vi "nanocal -- nuclear schottky fit V3.vi"() -> ()   [LabVIEW 2020] (continued)
\"mm1\"-> 0.000103608352  , \"mm2\"-> 0.017542867394  , \"mm3\"-> 0.085978401835  , \"T\"->  0.300000000000  , \"B\"-> 12.000000000000  , \"θ\"-> 90.000000000000  |>   , \r76 ->   <| \"ζ\"->  0.044154556051  , \"τ1\"-> 0.038823125235  , \"τS\"-> 0.027069314930  , \"τN\"-> 0.013601990730  , \"τC\"-> 0.002287979276  , \"κ0\"-> 0.000000002359  , \"mm1\"-> 0.000089763345  , \"mm2\"-> 0.018083678254  , \"mm3\"-> 0.065404792018  , \"T\"->  0.360000000000  , \"B\"-> 12.000000000000  , \"θ\"-> 90.000000000000  |>   , \r77 ->   <| \"ζ\"->  0.032748569996  , \"τ1\"-> 0.031072007290  , \"τS\"-> 0.024343937548  , \"τN\"-> 0.006961654481  , \"τC\"-> 0.002967111565  , \"κ0\"-> 0.000000002964  , \"mm1\"-> 0.000084402249  , \"mm2\"-> 0.018055855929  , \"mm3\"-> 0.048229666078  , \"T\"->  0.430000000000  , \"B\"-> 12.000000000000  , \"θ\"-> 90.000000000000  |>   , \r78 ->   <| \"ζ\"->  0.027599263457  , \"τ1\"-> 0.026239105728  , \"τS\"-> 0.022370859308  , \"τN\"-> 0.003857632966  , \"τC\"-> 0.003499360499  , \"κ0\"-> 0.000000003681  , \"mm1\"-> 0.000081816106  , \"mm2\"-> 0.017901054668  , \"mm3\"-> 0.038707974796  , \"T\"->  0.512000000000  , \"B\"-> 12.000000000000  , \"θ\"-> 90.000000000000  |>   , \r79 ->   <| \"ζ\"->  0.020568815513  , \"τ1\"-> 0.023045965648  , \"τS\"-> 0.020791387386  , \"τN\"-> 0.002229171297  , \"τC\"-> 0.004427475438  , \"κ0\"-> 0.000000004398  , \"mm1\"-> 0.000074037290  , \"mm2\"-> 0.017820522459  , \"mm3\"-> 0.033072945644  , \"T\"->  0.610000000000  , \"B\"-> 12.000000000000  , \"θ\"-> 90.000000000000  |>   , \r80 ->   <| \"ζ\"->  0.016159836955  , \"τ1\"-> 0.019958638777  , \"τS\"-> 0.018730096307  , \"τN\"-> 0.000899236968  , \"τC\"-> 0.005152267403  , \"κ0\"-> 0.000000006087  , \"mm1\"-> 0.000064651231  , \"mm2\"-> 0.017530317649  , \"mm3\"-> 0.027462477400  , \"T\"->  0.810000000000  , \"B\"-> 12.000000000000  , \"θ\"-> 90.000000000000  |>   , \r81 ->   <| \"ζ\"->  0.014495870556  , \"τ1\"-> 0.019990087457  , \"τS\"-> 0.016832201384  , \"τN\"-> 0.000455517238  , \"τC\"-> 0.005555782498  , \"κ0\"-> 0.000000008420  , \"mm1\"-> 0.000060055560  , \"mm2\"-> 0.018114231010  , \"mm3\"-> 0.024909902538  , \"T\"->  1.100000000000  , \"B\"-> 12.000000000000  , \"θ\"-> 90.000000000000  |>   , \r82 ->   <| \"ζ\"->  0.014043763709  , \"τ1\"-> 0.018292068543  , \"τS\"-> 0.011311396743  , \"τN\"-> 0.000128802259  , \"τC\"-> 0.008087849636  , \"κ0\"-> 0.000000014258  , \"mm1\"-> 0.000065912054  , \"mm2\"-> 0.017276417784  , \"mm3\"-> 0.020638450794  , \"T\"->  1.800000000000  , \"B\"-> 12.000000000000  , \"θ\"-> 90.000000000000  |>   , \r83 ->   <| \"ζ\"->  0.016187684631  , \"τ1\"-> 0.018325345271  , \"τS\"-> 0.007510087776  , \"τN\"-> 0.000028419157  , \"τC\"-> 0.008115463080  , \"κ0\"-> 0.000000024747  , \"mm1\"-> 0.000062903858  , \"mm2\"-> 0.015524812312  , \"mm3\"-> 0.018513630087  , \"T\"->  3.000000000000  , \"B\"-> 12.000000000000  , \"θ\"-> 90.000000000000  |>   , \r84 ->   <| \"ζ\"->  0.027897403691  , \"τ1\"-> 0.014639690770  , \"τS\"-> 0.004105291179  , \"τN\"-> 0.000006999171  , \"τC\"-> 0.007414449545  , \"κ0\"-> 0.000000059701  , \"mm1\"-> 0.000073450671  , \"mm2\"-> 0.011534391407  , \"mm3\"-> 0.014673310811  , \"T\"->  5.700000000000  , \"B\"-> 12.000000000000  , \"θ\"-> 90.000000000000  |>   , \r"
  out "filenames":map{i32, string}(c390)={4026="CeCoIn5_3rd_4026_ref_12T_0.127K_60deg_changeT_fsweep_labview_.dat", 4027="CeCoIn5_3rd_4027_ref_12T_0.15K_60deg_changeT_fsweep_labview_.dat", 4028="CeCoIn5_3rd_4028_ref_12T_0.179K_60deg_changeT_fsweep_labview_.dat", 4029="CeCoIn5_3rd_4029_ref_12T_0.20K_60deg_changeT_fsweep_labview_.dat", 4030="CeCoIn5_3rd_4030_ref_12T_0.24K_60deg_changeT_fsweep_labview_.dat", 4031="CeCoIn5_3rd_4031_ref_12T_0.287K_60deg_changeT_fsweep_labview_.dat", 4032="CeCoIn5_3rd_4032_ref_12T_0.33K_60deg_changeT_fsweep_labview_.dat", 4033="CeCoIn5_3rd_4033_ref_12T_0.43K_60deg_changeT_fsweep_labview_.dat", 4034="CeCoIn5_3rd_4034_ref_12T_0.51K_60deg_changeT_fsweep_labview_.dat", 4035="CeCoIn5_3rd_4035_ref_12T_0.62K_60deg_changeT_fsweep_labview_.dat", 4036="CeCoIn5_3rd_4036_ref_12T_0.83K_60deg_changeT_fsweep_labview_.dat", 4037="CeCoIn5_3rd_4037_ref_12T_1.13K_60deg_changeT_fsweep_labview_.dat", 4038="CeCoIn5_3rd_4038_ref_12T_1.90K_60deg_changeT_fsweep_labview_.dat", 4039="CeCoIn5_3rd_4039_ref_12T_3.15K_60deg_changeT_fsweep_labview_.dat", 4040="CeCoIn5_3rd_4040_ref_12T_5.70K_60deg_changeT_fsweep_labview_.dat", 4041="CeCoIn5_3rd_4041_ref_12T_7.87K_60deg_changeT_fsweep_labview_.dat", 4042="CeCoIn5_3rd_4042_ref_12T_9.80K_60deg_changeT_fsweep_labview_.dat", 4043="CeCoIn5_3rd_4043_ref_12T_12.36K_60deg_changeT_fsweep_labview_.dat", 4044="CeCoIn5_3rd_4044_ref_12T_14.80K_60deg_changeT_fsweep_labview_.dat", 4045="CeCoIn5_3rd_4045_ref_12T_16.42K_60deg_changeT_fsweep_labview_.dat", 4046="CeCoIn5_3rd_4046_ref_12T_18.04K_60deg_changeT_fsweep_labview_.dat", 4047="CeCoIn5_2nd_4047_12T_ref_0.14K_0deg_changeT_fsweep_labview_.dat", 4048="CeCoIn5_2nd_4048_12T_ref_0.17K_0deg_changeT_fsweep_labview_.dat", 4049="CeCoIn5_2nd_4049_12T_ref_0.20K_0deg_changeT_fsweep_labview_.dat", 4050="CeCoIn5_2nd_4050_12T_ref_0.22K_0deg_changeT_fsweep_labview_.dat", 4051="CeCoIn5_2nd_4051_12T_ref_0.28K_0deg_changeT_fsweep_labview_.dat", 4052="CeCoIn5_2nd_4052_12T_ref_0.33K_0deg_changeT_fsweep_labview_.dat", 4053="CeCoIn5_2nd_4053_12T_ref_0.40K_0deg_changeT_fsweep_labview_.dat", 4054="CeCoIn5_2nd_4054_12T_ref_0.48K_0deg_changeT_fsweep_labview_.dat", 4055="CeCoIn5_2nd_4055_12T_ref_0.58K_0deg_changeT_fsweep_labview_.dat", 4056="CeCoIn5_2nd_4056_12T_ref_0.68K_0deg_changeT_fsweep_labview_.dat", 4057="CeCoIn5_2nd_4057_12T_ref_0.91K_0deg_changeT_fsweep_labview_.dat", 4058="CeCoIn5_2nd_4058_12T_ref_1.23K_0deg_changeT_fsweep_labview_.dat", 4059="CeCoIn5_2nd_4059_12T_ref_1.97K_0deg_changeT_fsweep_labview_.dat", 4060="CeCoIn5_2nd_4060_12T_ref_3.19K_0deg_changeT_fsweep_labview_.dat", 4061="CeCoIn5_2nd_4061_12T_ref_5.82K_0deg_changeT_fsweep_labview_.dat", 4070="CeCoIn5_2nd_4070_12T_ref_0.20K_90deg_changeT_fsweep_labview_.dat", 4071="CeCoIn5_2nd_4071_12T_ref_0.14K_90deg_changeT_fsweep_labview_.dat", 4072="CeCoIn5_2nd_4072_12T_ref_0.18K_90deg_changeT_fsweep_labview_.dat", 4073="CeCoIn5_2nd_4073_12T_ref_0.22K_90deg_changeT_fsweep_labview_.dat", 4074="CeCoIn5_2nd_4074_12T_ref_0.27K_90deg_changeT_fsweep_labview_.dat", 4075="CeCoIn5_2nd_4075_12T_ref_0.33K_90deg_changeT_fsweep_labview_.dat", 4076="CeCoIn5_2nd_4076_12T_ref_0.39K_90deg_changeT_fsweep_labview_.dat", 4077="CeCoIn5_2nd_4077_12T_ref_0.48K_90deg_changeT_fsweep_labview_.dat", 4078="CeCoIn5_2nd_4078_12T_ref_0.58K_90deg_changeT_fsweep_labview_.dat", 4079="CeCoIn5_2nd_4079_12T_ref_0.68K_90deg_changeT_fsweep_labview_.dat", 4080="CeCoIn5_2nd_4080_12T_ref_0.91K_90deg_changeT_fsweep_labview_.dat", 4081="CeCoIn5_2nd_4081_12T_ref_1.23K_90deg_changeT_fsweep_labview_.dat", 4082="CeCoIn5_2nd_4082_12T_ref_2.05K_90deg_changeT_fsweep_labview_.dat", 4083="CeCoIn5_2nd_4083_12T_ref_3.31K_90deg_changeT_fsweep_labview_.dat", 4084="CeCoIn5_2nd_4084_12T_ref_6.0K_90deg_changeT_fsweep_labview_.dat", 4094="CeCoIn5_2nd_4094_6T_0.30K_90deg_ref_changeB_fsweep_labview_.dat", 4095="CeCoIn5_2nd_4095_6T_0.197K_90deg_ref_changeB_fsweep_labview_.dat", 4098="CeCoIn5_2nd_4098_6T_0.148K_90deg_ref_changeB_fsweep_labview_.dat", 4099="CeCoIn5_2nd_4099_9T_0.197K_90deg_ref_changeB_fsweep_labview_.dat", 4100="CeCoIn5_2nd_4100_11T_0.197K_90deg_ref_changeB_fsweep_labview_.dat", 4101="CeCoIn5_2nd_4101_10T_0.197K_90deg_ref_changeB_fsweep_labview_.dat", 4102="CeCoIn5_2nd_4102_8T_0.197K_90deg_ref_changeB_fsweep_labview_.dat", 4103="CeCoIn5_2nd_4103_7T_0.197K_90deg_ref_changeB_fsweep_labview_.dat", 4104="CeCoIn5_2nd_4104_5T_0.197K_90deg_ref_changeB_fsweep_labview_.dat", 4105="CeCoIn5_2nd_4105_0T_0.197K_90deg_ref_changeB_fsweep_labview_.dat", 4106="CeCoIn5_2nd_4106_0T_1.55K_90deg_ref_changeB_fsweep_labview_.dat", 4107="CeCoIn5_2nd_4107_0T_1.00K_90deg_ref_changeB_fsweep_labview_.dat", 4108="CeCoIn5_2nd_4108_0T_0.67K_90deg_ref_changeB_fsweep_labview_.dat", 4110="CeCoIn5_4th_4110_ref_12T_0.16K_30deg_changeT_fsweep_labview_.dat", 4112="CeCoIn5_4th_4112_ref_12T_0.17K_30deg_changeT_fsweep_labview_.dat", 4113="CeCoIn5_4th_4113_ref_12T_0.14K_30deg_changeT_fsweep_labview_.dat", 4114="CeCoIn5_4th_4114_ref_12T_0.20K_30deg_changeT_fsweep_labview_.dat", 4115="CeCoIn5_4th_4115_ref_12T_0.25K_30deg_changeT_fsweep_labview_.dat", 4116="CeCoIn5_4th_4116_ref_12T_0.30K_30deg_changeT_fsweep_labview_.dat", 4117="CeCoIn5_4th_4117_ref_12T_0.36K_30deg_changeT_fsweep_labview_.dat", 4118="CeCoIn5_4th_4118_ref_12T_0.43K_30deg_changeT_fsweep_labview_.dat", 4119="CeCoIn5_4th_4119_ref_12T_0.53K_30deg_changeT_fsweep_labview_.dat", 4120="CeCoIn5_4th_4120_ref_12T_0.62K_30deg_changeT_fsweep_labview_.dat", 4121="CeCoIn5_4th_4121_ref_12T_0.83K_30deg_changeT_fsweep_labview_.dat", 4122="CeCoIn5_4th_4122_ref_12T_1.13K_30deg_changeT_fsweep_labview_.dat", 4123="CeCoIn5_4th_4123_ref_12T_1.90K_30deg_changeT_fsweep_labview_.dat", 4124="CeCoIn5_4th_4124_ref_12T_3.10K_30deg_changeT_fsweep_labview_.dat", 8026="CeCoIn5_3rd_8026_sam_12T_0.127K_60deg_changeT_fsweep_labview_.dat", 8027="CeCoIn5_3rd_8027_sam_12T_0.15K_60deg_changeT_fsweep_labview_.dat", 8028="CeCoIn5_3rd_8028_sam_12T_0.179K_60deg_changeT_fsweep_labview_.dat", 8029="CeCoIn5_3rd_8029_sam_12T_0.20K_60deg_changeT_fsweep_labview_.dat", 8030="CeCoIn5_3rd_8030_sam_12T_0.24K_60deg_changeT_fsweep_labview_.dat", 8031="CeCoIn5_3rd_8031_sam_12T_0.287K_60deg_changeT_fsweep_labview_.dat", 8032="CeCoIn5_3rd_8032_sam_12T_0.33K_60deg_changeT_fsweep_labview_.dat", 8033="CeCoIn5_3rd_8033_sam_12T_0.43K_60deg_changeT_fsweep_labview_.dat", 8034="CeCoIn5_3rd_8034_sam_12T_0.51K_60deg_changeT_fsweep_labview_.dat", 8035="CeCoIn5_3rd_8035_sam_12T_0.62K_60deg_changeT_fsweep_labview_.dat", 8036="CeCoIn5_3rd_8036_sam_12T_0.83K_60deg_changeT_fsweep_labview_.dat", 8037="CeCoIn5_3rd_8037_sam_12T_1.13K_60deg_changeT_fsweep_labview_.dat", 8038="CeCoIn5_3rd_8038_sam_12T_1.90K_60deg_changeT_fsweep_labview_.dat", 8039="CeCoIn5_3rd_8039_sam_12T_3.15K_60deg_changeT_fsweep_labview_.dat", 8040="CeCoIn5_3rd_8040_sam_12T_5.70K_60deg_changeT_fsweep_labview_.dat", 8041="CeCoIn5_3rd_8041_sam_12T_7.87K_60deg_changeT_fsweep_labview_.dat", 8042="CeCoIn5_3rd_8042_sam_12T_9.80K_60deg_changeT_fsweep_labview_.dat", 8043="CeCoIn5_3rd_8043_sam_12T_12.36K_60deg_changeT_fsweep_labview_.dat", 8044="CeCoIn5_3rd_8044_sam_12T_14.80K_60deg_changeT_fsweep_labview_.dat", 8045="CeCoIn5_3rd_8045_sam_12T_16.42K_60deg_changeT_fsweep_labview_.dat", 8046="CeCoIn5_3rd_8046_sam_12T_18.04K_60deg_changeT_fsweep_labview_.dat", 8047="CeCoIn5_2nd_8047_12T_sam_0.12K_0deg_changeT_fsweep_labview_.dat", 8048="CeCoIn5_2nd_8048_12T_sam_0.148K_0deg_changeT_fsweep_labview_.dat", 8049="CeCoIn5_2nd_8049_12T_sam_0.179K_0deg_changeT_fsweep_labview_.dat", 8050="CeCoIn5_2nd_8050_12T_sam_0.197K_0deg_changeT_fsweep_labview_.dat", 8051="CeCoIn5_2nd_8051_12T_sam_0.25K_0deg_changeT_fsweep_labview_.dat", 8052="CeCoIn5_2nd_8052_12T_sam_0.3K_0deg_changeT_fsweep_labview_.dat", 8053="CeCoIn5_2nd_8053_12T_sam_0.360K_0deg_changeT_fsweep_labview_.dat", 8054="CeCoIn5_2nd_8054_12T_sam_0.430K_0deg_changeT_fsweep_labview_.dat", 8055="CeCoIn5_2nd_8055_12T_sam_0.512K_0deg_changeT_fsweep_labview_.dat", 8056="CeCoIn5_2nd_8056_12T_sam_0.61K_0deg_changeT_fsweep_labview_.dat", 8057="CeCoIn5_2nd_8057_12T_sam_0.81K_0deg_changeT_fsweep_labview_.dat", 8058="CeCoIn5_2nd_8058_12T_sam_1.12K_0deg_changeT_fsweep_labview_.dat", 8059="CeCoIn5_2nd_8059_12T_sam_1.8K_0deg_changeT_fsweep_labview_.dat", 8060="CeCoIn5_2nd_8060_12T_sam_3.0K_0deg_changeT_fsweep_labview_.dat", 8061="CeCoIn5_2nd_8061_12T_sam_5.5K_0deg_changeT_fsweep_labview_.dat", 8070="CeCoIn5_2nd_8070_12T_sam_0.179K_90deg_changeT_fsweep_labview_.dat", 8071="CeCoIn5_2nd_8071_12T_sam_0.120K_90deg_changeT_fsweep_labview_.dat", 8072="CeCoIn5_2nd_8072_12T_sam_0.148K_90deg_changeT_fsweep_labview_.dat", 8073="CeCoIn5_2nd_8073_12T_sam_0.197K_90deg_changeT_fsweep_labview_.dat", 8074="CeCoIn5_2nd_8074_12T_sam_0.249K_90deg_changeT_fsweep_labview_.dat", 8075="CeCoIn5_2nd_8075_12T_sam_0.300K_90deg_changeT_fsweep_labview_.dat", 8076="CeCoIn5_2nd_8076_12T_sam_0.360K_90deg_changeT_fsweep_labview_.dat", 8077="CeCoIn5_2nd_8077_12T_sam_0.430K_90deg_changeT_fsweep_labview_.dat", 8078="CeCoIn5_2nd_8078_12T_sam_0.512K_90deg_changeT_fsweep_labview_.dat", 8079="CeCoIn5_2nd_8079_12T_sam_0.610K_90deg_changeT_fsweep_labview_.dat", 8080="CeCoIn5_2nd_8080_12T_sam_0.810K_90deg_changeT_fsweep_labview_.dat", 8081="CeCoIn5_2nd_8081_12T_sam_1.1K_90deg_changeT_fsweep_labview_.dat", 8082="CeCoIn5_2nd_8082_12T_sam_1.8K_90deg_changeT_fsweep_labview_.dat", 8083="CeCoIn5_2nd_8083_12T_sam_3.0K_90deg_changeT_fsweep_labview_.dat", 8084="CeCoIn5_2nd_8084_12T_sam_5.7K_90deg_changeT_fsweep_labview_.dat", 8094="CeCoIn5_2nd_8094_6T_0.30K_90deg_sam_changeB_fsweep_labview_.dat", 8095="CeCoIn5_2nd_8095_6T_0.197K_90deg_sam_changeB_fsweep_labview_.dat", 8098="CeCoIn5_2nd_8098_6T_0.148K_90deg_sam_changeB_fsweep_labview_.dat", 8099="CeCoIn5_2nd_8099_9T_0.197K_90deg_sam_changeB_fsweep_labview_.dat", 8100="CeCoIn5_2nd_8100_11T_0.197K_90deg_sam_changeB_fsweep_labview_.dat", 8101="CeCoIn5_2nd_8101_10T_0.197K_90deg_sam_changeB_fsweep_labview_.dat", 8102="CeCoIn5_2nd_8102_8T_0.197K_90deg_sam_changeB_fsweep_labview_.dat", 8103="CeCoIn5_2nd_8103_7T_0.197K_90deg_sam_changeB_fsweep_labview_.dat", 8104="CeCoIn5_2nd_8104_5T_0.197K_90deg_sam_changeB_fsweep_labview_.dat", 8105="CeCoIn5_2nd_8105_0T_0.197K_90deg_sam_changeB_fsweep_labview_.dat", 8106="CeCoIn5_2nd_8106_0T_1.55K_90deg_sam_changeB_fsweep_labview_.dat", 8107="CeCoIn5_2nd_8107_0T_1.00K_90deg_sam_changeB_fsweep_labview_.dat", 8108="CeCoIn5_2nd_8108_0T_0.67K_90deg_sam_changeB_fsweep_labview_.dat", 8110="CeCoIn5_4th_8110_sam_12T_0.16K_30deg_changeT_fsweep_labview_.dat", 8112="CeCoIn5_4th_8112_sam_12T_0.17K_30deg_changeT_fsweep_labview_.dat", 8113="CeCoIn5_4th_8113_sam_12T_0.14K_30deg_changeT_fsweep_labview_.dat", 8114="CeCoIn5_4th_8114_sam_12T_0.20K_30deg_changeT_fsweep_labview_.dat", 8115="CeCoIn5_4th_8115_sam_12T_0.25K_30deg_changeT_fsweep_labview_.dat", 8116="CeCoIn5_4th_8116_sam_12T_0.30K_30deg_changeT_fsweep_labview_.dat", 8117="CeCoIn5_4th_8117_sam_12T_0.36K_30deg_changeT_fsweep_labview_.dat", 8118="CeCoIn5_4th_8118_sam_12T_0.43K_30deg_changeT_fsweep_labview_.dat", 8119="CeCoIn5_4th_8119_sam_12T_0.53K_30deg_changeT_fsweep_labview_.dat", 8120="CeCoIn5_4th_8120_sam_12T_0.62K_30deg_changeT_fsweep_labview_.dat", 8121="CeCoIn5_4th_8121_sam_12T_0.83K_30deg_changeT_fsweep_labview_.dat", 8122="CeCoIn5_4th_8122_sam_12T_1.13K_30deg_changeT_fsweep_labview_.dat", 8123="CeCoIn5_4th_8123_sam_12T_1.90K_30deg_changeT_fsweep_labview_.dat", 8124="CeCoIn5_4th_8124_sam_12T_3.10K_30deg_changeT_fsweep_labview_.dat", 40047="CeCoIn5_3rd_40047_ref_12T_19.60K_60deg_changeT_fsweep_labview_.dat", 40049="CeCoIn5_3rd_40049_ref_12T_0.129K_60deg_changeT_fsweep_labview_.dat", 40125="CeCoIn5_4th___40125__(039)__C(f)_12T_0.157K_45deg _changeT_ref_fromraw__labview_.dat", 40126="CeCoIn5_4th___40126__(040)__C(f)_12T_0.120K_45deg_changeT_ref_fromraw__labview_.dat", 40127="CeCoIn5_4th___40127__(041)__C(f)_12T_0.170K_45deg_changeT_ref_fromraw__labview_.dat", 40128="CeCoIn5_4th___40128__(042)__C(f)_12T_0.200K_45deg_changeT_ref_fromraw__labview_.dat", 40129="CeCoIn5_4th___40129__(043)__C(f)_12T_0.255K_45deg_changeT_ref_fromraw__labview_.dat", 40130="CeCoIn5_4th___40130__(044)__C(f)_12T_0.300K_45deg_changeT_ref_fromraw__labview_.dat", 40131="CeCoIn5_4th___40131__(045)__C(f)_12T_0.360K_45deg_changeT_ref_fromraw__labview_.dat", 40132="CeCoIn5_4th___40132__(046)__C(f)_12T_0.43K_45deg_changeT_ref_fromraw__labview_.dat", 40133="CeCoIn5_4th___40133__(047)__C(f)_12T_0.53K_45deg_changeT_ref_fromraw__labview_.dat", 40134="CeCoIn5_4th___40134__(048)__C(f)_12T_0.62K_45deg_changeT_ref_fromraw__labview_.dat", 40135="CeCoIn5_4th___40135__(049)__C(f)_12T_0.83K_45deg_changeT_ref_fromraw__labview_.dat", 40136="CeCoIn5_4th___40136__(050)__C(f)_12T_1.13K_45deg_changeT_ref_fromraw__labview_.dat", 40137="CeCoIn5_4th___40137__(051)__C(f)_12T_1.90K_45deg_changeT_ref_fromraw__labview_.dat", 40138="CeCoIn5_4th___40138__(052)__C(f)_12T_3.10K_45deg_changeT_ref_fromraw__labview_.dat", 40139="CeCoIn5_4th___40139__(053)__C(f)_12T_5.70K_45deg_changeT_ref_fromraw__labview_.dat", 80047="CeCoIn5_3rd_80047_sam_12T_19.60K_60deg_changeT_fsweep_labview_.dat", 80049="CeCoIn5_3rd_80049_sam_12T_0.129K_60deg_changeT_fsweep_labview_.dat", 80125="CeCoIn5_4th___80125__(039)__C(f)_12T_0.157K_45deg _changeT_sam_fromraw__labview_.dat", 80126="CeCoIn5_4th___80126__(040)__C(f)_12T_0.120K_45deg_changeT_sam_fromraw__labview_.dat", 80127="CeCoIn5_4th___80127__(041)__C(f)_12T_0.170K_45deg_changeT_sam_fromraw__labview_.dat", 80128="CeCoIn5_4th___80128__(042)__C(f)_12T_0.200K_45deg_changeT_sam_fromraw__labview_.dat", 80129="CeCoIn5_4th___80129__(043)__C(f)_12T_0.255K_45deg_changeT_sam_fromraw__labview_.dat", 80130="CeCoIn5_4th___80130__(044)__C(f)_12T_0.300K_45deg_changeT_sam_fromraw__labview_.dat", 80131="CeCoIn5_4th___80131__(045)__C(f)_12T_0.360K_45deg_changeT_sam_fromraw__labview_.dat", 80132="CeCoIn5_4th___80132__(046)__C(f)_12T_0.43K_45deg_changeT_sam_fromraw__labview_.dat", 80133="CeCoIn5_4th___80133__(047)__C(f)_12T_0.53K_45deg_changeT_sam_fromraw__labview_.dat", 80134="CeCoIn5_4th___80134__(048)__C(f)_12T_0.62K_45deg_changeT_sam_fromraw__labview_.dat", 80135="CeCoIn5_4th___80135__(049)__C(f)_12T_0.83K_45deg_changeT_sam_fromraw__labview_.dat", 80136="CeCoIn5_4th___80136__(050)__C(f)_12T_1.13K_45deg_changeT_sam_fromraw__labview_.dat", 80137="CeCoIn5_4th___80137__(051)__C(f)_12T_1.90K_45deg_changeT_sam_fromraw__labview_.dat", 80138="CeCoIn5_4th___80138__(052)__C(f)_12T_3.10K_45deg_changeT_sam_fromraw__labview_.dat", 80139="CeCoIn5_4th___80139__(053)__C(f)_12T_5.70K_45deg_changeT_sam_fromraw__labview_.dat"}
  out "constrained filename lookup":map{i32, i32}(c390)={0=40126, 1=40125, 2=40127, 3=40128, 4=40129, 5=40130, 6=40131, 7=40132, 8=40133, 9=40134, 10=40135, 11=40136, 12=40137, 13=40138, 14=40139}
  out "Set of B's":set{dbl}(c389)={0.0, 5.0, 6.0, 7.0, 8.0, 9.0, 10.0, 11.0, 12.0}
  out "Set of θ's":set{dbl}(c389)={0.0, 30.0, 45.0, 60.0, 90.0}
  out "Set of T's":set{dbl}(c389)={0.12, 0.127, 0.129, 0.14, 0.148, 0.15, 0.157, 0.16, 0.17, 0.179, 0.18, 0.197, 0.2, 0.22, 0.24, 0.249, 0.25, 0.255, 0.27, 0.28, 0.287, 0.3, 0.33, 0.36, 0.39, 0.4, 0.43, 0.48, 0.51, 0.512, 0.53, 0.58, 0.61, 0.62, 0.67, 0.68, 0.81, 0.83, 0.91, 1.0, 1.1, 1.12, 1.13, 1.23, 1.55, 1.8, 1.9, 1.97, 2.05, 3.0, 3.1, 3.15, 3.19, 3.31, 5.5, 5.7, 5.82, 6.0, 7.87, 9.8, 12.36, 14.8, 16.42, 18.04, 19.6}
  out "B lookup":map{i32, dbl}(c390)={0=0.0, 1=5.0, 2=6.0, 3=7.0, 4=8.0, 5=9.0, 6=10.0, 7=11.0, 8=12.0}
  out "filesnames lookup":map{i32, i32}(c390)={0=8047, 1=8071, 2=40126, 3=80126, 4=4026, 5=8026, 6=40049, 7=80049, 8=4047, 9=4071, 10=4113, 11=8113, 12=4098, 13=8048, 14=8072, 15=8098, 16=4027, 17=8027, 18=40125, 19=80125, 20=4110, 21=8110, 22=4048, 23=4112, 24=8112, 25=40127, 26=80127, 27=4028, 28=8028, 29=8049, 30=8070, 31=4072, 32=4095, 33=4099, 34=4100, 35=4101, 36=4102, 37=4103, 38=4104, 39=4105, 40=8050, 41=8073, 42=8095, 43=8099, 44=8100, 45=8101, 46=8102, 47=8103, 48=8104, 49=8105, 50=4029, 51=4049, 52=4070, 53=4114, 54=8029, 55=8114, 56=40128, 57=80128, 58=4050, 59=4073, 60=4030, 61=8030, 62=8074, 63=4115, 64=8051, 65=8115, 66=40129, 67=80129, 68=4074, 69=4051, 70=4031, 71=8031, 72=4094, 73=4116, 74=8052, 75=8075, 76=8094, 77=8116, 78=40130, 79=80130, 80=4032, 81=4052, 82=4075, 83=8032, 84=4117, 85=8053, 86=8076, 87=8117, 88=40131, 89=80131, 90=4076, 91=4053, 92=4033, 93=4118, 94=8033, 95=8054, 96=8077, 97=8118, 98=40132, 99=80132, 100=4054, 101=4077, 102=4034, 103=8034, 104=8055, 105=8078, 106=4119, 107=8119, 108=40133, 109=80133, 110=4055, 111=4078, 112=8056, 113=8079, 114=4035, 115=4120, 116=8035, 117=8120, 118=40134, 119=80134, 120=4108, 121=8108, 122=4056, 123=4079, 124=8057, 125=8080, 126=4036, 127=4121, 128=8036, 129=8121, 130=40135, 131=80135, 132=4057, 133=4080, 134=4107, 135=8107, 136=8081, 137=8058, 138=4037, 139=4122, 140=8037, 141=8122, 142=40136, 143=80136, 144=4058, 145=4081, 146=4106, 147=8106, 148=8059, 149=8082, 150=4038, 151=4123, 152=8038, 153=8123, 154=40137, 155=80137, 156=4059, 157=4082, 158=8060, 159=8083, 160=4124, 161=8124, 162=40138, 163=80138, 164=4039, 165=8039, 166=4060, 167=4083, 168=8061, 169=4040, 170=8040, 171=8084, 172=40139, 173=80139, 174=4061, 175=4084, 176=4041, 177=8041, 178=4042, 179=8042, 180=4043, 181=8043, 182=4044, 183=8044, 184=4045, 185=8045, 186=4046, 187=8046, 188=40047, 189=80047}
  out "θ lookup":map{i32, dbl}(c390)={0=0.0, 1=30.0, 2=45.0, 3=60.0, 4=90.0}
  out "T lookup":map{i32, dbl}(c390)={0=0.12, 1=0.127, 2=0.129, 3=0.14, 4=0.148, 5=0.15, 6=0.157, 7=0.16, 8=0.17, 9=0.179, 10=0.18, 11=0.197, 12=0.2, 13=0.22, 14=0.24, 15=0.249, 16=0.25, 17=0.255, 18=0.27, 19=0.28, 20=0.287, 21=0.3, 22=0.33, 23=0.36, 24=0.39, 25=0.4, 26=0.43, 27=0.48, 28=0.51, 29=0.512, 30=0.53, 31=0.58, 32=0.61, 33=0.62, 34=0.67, 35=0.68, 36=0.81, 37=0.83, 38=0.91, 39=1.0, 40=1.1, 41=1.12, 42=1.13, 43=1.23, 44=1.55, 45=1.8, 46=1.9, 47=1.97, 48=2.05, 49=3.0, 50=3.1, 51=3.15, 52=3.19, 53=3.31, 54=5.5, 55=5.7, 56=5.82, 57=6.0, 58=7.87, 59=9.8, 60=12.36, 61=14.8, 62=16.42, 63=18.04, 64=19.6}
  out "Set of Sides":set{dbl}(c389)={4000.0, 8000.0}
  out "Side lookup":map{i32, dbl}(c390)={0=4000.0, 1=8000.0}
  out "Set of Change":set{dbl}(c389)={1.0, 2.0}
  out "change lookup":map{i32, dbl}(c390)={0=1.0, 1=2.0}
  out "backup mathematica string OUT backup":string="  48 ->   <| \"ζ\"-> 0.225182112153  , \"τ1\"-> 0.030427185371  , \"τS\"-> 0.215756406989  , \"τN\"-> 0.297516075068  , \"τC\"-> 0.001159880124  , \"κ0\"-> 0.000000000757  , \"T\"-> 0.148000000000  , \"mm1\"-> 0.000000000000  , \"mm2\"-> 0.000000000000  , \"mm3\"-> 0.000000000000  , \"θ\"-> 0.000000000000  |>   , \r49 ->   <| \"ζ\"-> 0.172076901868  , \"τ1\"-> 0.029034369734  , \"τS\"-> 0.155813864567  , \"τN\"-> 0.144653734876  , \"τC\"-> 0.001114471886  , \"κ0\"-> 0.000000001041  , \"T\"-> 0.179000000000  , \"mm1\"-> 0.000000000000  , \"mm2\"-> 0.000000000000  , \"mm3\"-> 0.000000000000  , \"θ\"-> 0.000000000000  |>   , \r50 ->   <| \"ζ\"-> 0.148077728243  , \"τ1\"-> 0.028544607399  , \"τS\"-> 0.124620640187  , \"τN\"-> 0.093757074751  , \"τC\"-> 0.001082877171  , \"κ0\"-> 0.000000001180  , \"T\"-> 0.197000000000  , \"mm1\"-> 0.000000000000  , \"mm2\"-> 0.000000000000  , \"mm3\"-> 0.000000000000  , \"θ\"-> 0.000000000000  |>   , \r51 ->   <| \"ζ\"-> 0.081193222097  , \"τ1\"-> 0.024715806431  , \"τS\"-> 0.089455978355  , \"τN\"-> 0.032053841538  , \"τC\"-> 0.001544599185  , \"κ0\"-> 0.000000001536  , \"T\"-> 0.250000000000  , \"mm1\"-> 0.000000000000  , \"mm2\"-> 0.000000000000  , \"mm3\"-> 0.000000000000  , \"θ\"-> 0.000000000000  |>   , \r52 ->   <| \"ζ\"-> 0.048082496373  , \"τ1\"-> 0.022642786515  , \"τS\"-> 0.068869549235  , \"τN\"-> 0.016486235683  , \"τC\"-> 0.002476229885  , \"κ0\"-> 0.000000001973  , \"T\"-> 0.300000000000  , \"mm1\"-> 0.000000000000  , \"mm2\"-> 0.000000000000  , \"mm3\"-> 0.000000000000  , \"θ\"-> 0.000000000000  |>   , \r53 ->   <| \"ζ\"-> 0.038407326202  , \"τ1\"-> 0.020371560008  , \"τS\"-> 0.055508745241  , \"τN\"-> 0.008451508810  , \"τC\"-> 0.002530832197  , \"κ0\"-> 0.000000002423  , \"T\"-> 0.360000000000  , \"mm1\"-> 0.000000000000  , \"mm2\"-> 0.000000000000  , \"mm3\"-> 0.000000000000  , \"θ\"-> 0.000000000000  |>   , \r54 ->   <| \"ζ\"-> 0.025817013343  , \"τ1\"-> 0.018385471103  , \"τS\"-> 0.045747558757  , \"τN\"-> 0.005165003032  , \"τC\"-> 0.002680275541  , \"κ0\"-> 0.000000002982  , \"T\"-> 0.430000000000  , \"mm1\"-> 0.000000000000  , \"mm2\"-> 0.000000000000  , \"mm3\"-> 0.000000000000  , \"θ\"-> 0.000000000000  |>   , \r55 ->   <| \"ζ\"-> 0.019908376980  , \"τ1\"-> 0.016902177597  , \"τS\"-> 0.037431350421  , \"τN\"-> 0.003115611581  , \"τC\"-> 0.002813000351  , \"κ0\"-> 0.000000003723  , \"T\"-> 0.512000000000  , \"mm1\"-> 0.000000000000  , \"mm2\"-> 0.000000000000  , \"mm3\"-> 0.000000000000  , \"θ\"-> 0.000000000000  |>   , \r56 ->   <| \"ζ\"-> 0.018376000000  , \"τ1\"-> 0.014989979497  , \"τS\"-> 0.031364970092  , \"τN\"-> 0.001876083588  , \"τC\"-> 0.004034409107  , \"κ0\"-> 0.000000004410  , \"T\"-> 0.610000000000  , \"mm1\"-> 0.000000000000  , \"mm2\"-> 0.000000000000  , \"mm3\"-> 0.000000000000  , \"θ\"-> 0.000000000000  |>   , \r57 ->   <| \"ζ\"-> 0.015651665128  , \"τ1\"-> 0.013298894889  , \"τS\"-> 0.022882494925  , \"τN\"-> 0.000826522678  , \"τC\"-> 0.005306542804  , \"κ0\"-> 0.000000006075  , \"T\"-> 0.810000000000  , \"mm1\"-> 0.000000000000  , \"mm2\"-> 0.000000000000  , \"mm3\"-> 0.000000000000  , \"θ\"-> 0.000000000000  |>   , \r58 ->   <| \"ζ\"-> 0.011916480594  , \"τ1\"-> 0.012551282481  , \"τS\"-> 0.018233218660  , \"τN\"-> 0.000345702746  , \"τC\"-> 0.004699451527  , \"κ0\"-> 0.000000008451  , \"T\"-> 1.120000000000  , \"mm1\"-> 0.000000000000  , \"mm2\"-> 0.000000000000  , \"mm3\"-> 0.000000000000  , \"θ\"-> 0.000000000000  |>   , \r59 ->   <| \"ζ\"-> 0.012831327568  , \"τ1\"-> 0.013315909415  , \"τS\"-> 0.012590836847  , \"τN\"-> 0.000065003013  , \"τC\"-> 0.005276356243  , \"κ0\"-> 0.000000013610  , \"T\"-> 1.800000000000  , \"mm1\"-> 0.000000000000  , \"mm2\"-> 0.000000000000  , \"mm3\"-> 0.000000000000  , \"θ\"-> 0.000000000000  |>   , \r60 ->   <| \"ζ\"-> 0.019774146838  , \"τ1\"-> 0.013257273421  , \"τS\"-> 0.007064131508  , \"τN\"-> 0.000028000819  , \"τC\"-> 0.006942241845  , \"κ0\"-> 0.000000023477  , \"T\"-> 3.000000000000  , \"mm1\"-> 0.000000000000  , \"mm2\"-> 0.000000000000  , \"mm3\"-> 0.000000000000  , \"θ\"-> 0.000000000000  |>   , \r61 ->   <| \"ζ\"-> 0.029251354442  , \"τ1\"-> 0.014634751206  , \"τS\"-> 0.003873958746  , \"τN\"-> 0.000007000487  , \"τC\"-> 0.006827504775  , \"κ0\"-> 0.000000056438  , \"T\"-> 5.500000000000  , \"mm1\"-> 0.000000000000  , \"mm2\"-> 0.000000000000  , \"mm3\"-> 0.000000000000  , \"θ\"-> 0.000000000000  |>   , \r70 ->   <| \"ζ\"-> 0.160286026344  , \"τ1\"-> 0.073452047785  , \"τS\"-> 0.044872374187  , \"τN\"-> 0.162076895387  , \"τC\"-> 0.001481759328  , \"κ0\"-> 0.000000001039  , \"T\"-> 0.179000000000  , \"mm1\"-> 0.000000000000  , \"mm2\"-> 0.000000000000  , \"mm3\"-> 0.000000000000  , \"θ\"-> 90.000000000000  |>   , \r71 ->   <| \"ζ\"-> 0.317192968490  , \"τ1\"-> 0.095324848000  , \"τS\"-> 0.087097785701  , \"τN\"-> 0.936221653169  , \"τC\"-> 0.001480807262  , \"κ0\"-> 0.000000000534  , \"T\"-> 0.120000000000  , \"mm1\"-> 0.000000000000  , \"mm2\"-> 0.000000000000  , \"mm3\"-> 0.000000000000  , \"θ\"-> 90.000000000000  |>   , \r72 ->   <| \"ζ\"-> 0.222764630124  , \"τ1\"-> 0.096058032825  , \"τS\"-> 0.066495942806  , \"τN\"-> 0.366151877245  , \"τC\"-> 0.001319275999  , \"κ0\"-> 0.000000000769  , \"T\"-> 0.148000000000  , \"mm1\"-> 0.000000000000  , \"mm2\"-> 0.000000000000  , \"mm3\"-> 0.000000000000  , \"θ\"-> 90.000000000000  |>   , \r73 ->   <| \"ζ\"-> 0.136082903087  , \"τ1\"-> 0.070214285183  , \"τS\"-> 0.041562366618  , \"τN\"-> 0.122478563978  , \"τC\"-> 0.001561716081  , \"κ0\"-> 0.000000001214  , \"T\"-> 0.197000000000  , \"mm1\"-> 0.000000000000  , \"mm2\"-> 0.000000000000  , \"mm3\"-> 0.000000000000  , \"θ\"-> 90.000000000000  |>   , \r74 ->   <| \"ζ\"-> 0.079924133870  , \"τ1\"-> 0.053892600038  , \"τS\"-> 0.033721986821  , \"τN\"-> 0.048194390820  , \"τC\"-> 0.001786420268  , \"κ0\"-> 0.000000001543  , \"T\"-> 0.249000000000  , \"mm1\"-> 0.000000000000  , \"mm2\"-> 0.000000000000  , \"mm3\"-> 0.000000000000  , \"θ\"-> 90.000000000000  |>   , \r75 ->   <| \"ζ\"-> 0.055680730504  , \"τ1\"-> 0.044845519236  , \"τS\"-> 0.029550773155  , \"τN\"-> 0.023428217313  , \"τC\"-> 0.002197475136  , \"κ0\"-> 0.000000001960  , \"T\"-> 0.300000000000  , \"mm1\"-> 0.000000000000  , \"mm2\"-> 0.000000000000  , \"mm3\"-> 0.000000000000  , \"θ\"-> 90.000000000000  |>   , \r76 ->   <| \"ζ\"-> 0.040648812263  , \"τ1\"-> 0.038083560479  , \"τS\"-> 0.026574795079  , \"τN\"-> 0.013361826633  , \"τC\"-> 0.002899405432  , \"κ0\"-> 0.000000002383  , \"T\"-> 0.360000000000  , \"mm1\"-> 0.000000000000  , \"mm2\"-> 0.000000000000  , \"mm3\"-> 0.000000000000  , \"θ\"-> 90.000000000000  |>   , \r77 ->   <| \"ζ\"-> 0.031873906103  , \"τ1\"-> 0.030223838950  , \"τS\"-> 0.024286132427  , \"τN\"-> 0.006926780152  , \"τC\"-> 0.002978043437  , \"κ0\"-> 0.000000002967  , \"T\"-> 0.430000000000  , \"mm1\"-> 0.000000000000  , \"mm2\"-> 0.000000000000  , \"mm3\"-> 0.000000000000  , \"θ\"-> 90.000000000000  |>   , \r78 ->   <| \"ζ\"-> 0.025948172116  , \"τ1\"-> 0.025051552712  , \"τS\"-> 0.022571188655  , \"τN\"-> 0.003812228812  , \"τC\"-> 0.003259730052  , \"κ0\"-> 0.000000003686  , \"T\"-> 0.512000000000  , \"mm1\"-> 0.000000000000  , \"mm2\"-> 0.000000000000  , \"mm3\"-> 0.000000000000  , \"θ\"-> 90.000000000000  |>   , \r79 ->   <| \"ζ\"-> 0.020946044060  , \"τ1\"-> 0.024756174566  , \"τS\"-> 0.021099556284  , \"τN\"-> 0.002276701384  , \"τC\"-> 0.004159440288  , \"κ0\"-> 0.000000004389  , \"T\"-> 0.610000000000  , \"mm1\"-> 0.000000000000  , \"mm2\"-> 0.000000000000  , \"mm3\"-> 0.000000000000  , \"θ\"-> 90.000000000000  |>   , \r80 ->   <| \"ζ\"-> 0.014774082145  , \"τ1\"-> 0.015773102766  , \"τS\"-> 0.018723894921  , \"τN\"-> 0.000790199963  , \"τC\"-> 0.005097561693  , \"κ0\"-> 0.000000006095  , \"T\"-> 0.810000000000  , \"mm1\"-> 0.000000000000  , \"mm2\"-> 0.000000000000  , \"mm3\"-> 0.000000000000  , \"θ\"-> 90.000000000000  |>   , \r81 ->   <| \"ζ\"-> 0.013971175207  , \"τ1\"-> 0.015831825440  , \"τS\"-> 0.017293056061  , \"τN\"-> 0.000406001835  , \"τC\"-> 0.005061653181  , \"κ0\"-> 0.000000008423  , \"T\"-> 1.100000000000  , \"mm1\"-> 0.000000000000  , \"mm2\"-> 0.000000000000  , \"mm3\"-> 0.000000000000  , \"θ\"-> 90.000000000000  |>   , \r82 ->   <| \"ζ\"-> 0.014703834330  , \"τ1\"-> 0.019025451961  , \"τS\"-> 0.011790469569  , \"τN\"-> 0.000107003492  , \"τC\"-> 0.007625608278  , \"κ0\"-> 0.000000014259  , \"T\"-> 1.800000000000  , \"mm1\"-> 0.000000000000  , \"mm2\"-> 0.000000000000  , \"mm3\"-> 0.000000000000  , \"θ\"-> 90.000000000000  |>   , \r83 ->   <| \"ζ\"-> 0.021950059397  , \"τ1\"-> 0.019029879523  , \"τS\"-> 0.006582834729  , \"τN\"-> 0.000028012011  , \"τC\"-> 0.009051896214  , \"κ0\"-> 0.000000024750  , \"T\"-> 3.000000000000  , \"mm1\"-> 0.000000000000  , \"mm2\"-> 0.000000000000  , \"mm3\"-> 0.000000000000  , \"θ\"-> 90.000000000000  |>   , \r84 ->   <| \"ζ\"-> 0.027897403691  , \"τ1\"-> 0.014639690770  , \"τS\"-> 0.004105291179  , \"τN\"-> 0.000006999171  , \"τC\"-> 0.007414449545  , \"κ0\"-> 0.000000059701  , \"T\"-> 5.700000000000  , \"mm1\"-> 0.000073450671  , \"mm2\"-> 0.014673310812  , \"mm3\"-> 0.011534391407  , \"θ\"-> 90.000000000000  |>   , \r"
  in  "generate empty string from filelist":bool
  in  "tr":T3=enum."add - ω"
  in  "generate labview files":bool
  in  "string notes":string="\"T\"-> 0.225000,    \"ζ\"-> 0.006057  , \"τ1\"-> 0.011106  , \"τS\"-> 0.134857  , \"τN\"-> 0.000042  , \"τC\"-> 0.012982  , \"κ0\"-> 0.000000101776  , \"mm1\"-> 0.000071  , \"mm2\"-> 0.148631  , \"mm3\"-> 0.011103 "
  in  "load! :l":bool
  in  "Read from file":path=path "/opt/new/Dropbox/shared_AkashAndreas/paper-CeCoIn5/dataset--changeT--12T--0deg--60deg--90deg/CeCoIn5_4th___40126__(040)__C(f)_12T_0.120K_45deg_changeT_ref_fromraw__labview_.dat"
  in  "parse! :p":bool
  in  "String":string=" <| \"ζ\"->  0.556029763285  , \"τ1\"-> 0.055218717016  , \"τS\"-> 0.175069136234  , \"τN\"-> 0.345483484638  , \"τC\"-> 0.000911255863  , \"κ0\"-> 0.000000000418  , \"mm1\"-> 0.000000000000  , \"mm2\"-> 0.000000000000  , \"mm3\"-> 0.000000000000  , \"T\"->  0.120000000000  , \"B\"-> 12.000000000000  , \"θ\"-> 45.000000000000  |> "
  in  "backup string :b":string=" <| \"ζ\"->  0.167234158379  , \"τ1\"-> 0.020665214756  , \"τS\"-> 0.072250691270  , \"τN\"-> 0.020708769022  , \"τC\"-> 0.001243822553  , \"κ0\"-> 0.000000001059  , \"mm1\"-> 0.000000000000  , \"mm2\"-> 0.000000000000  , \"mm3\"-> 0.000000000000  , \"T\"->  5.700000000000  , \"B\"-> 12.000000000000  , \"θ\"-> 45.000000000000  |> "
  in  "plots":enum32{"Page 1", "Page 2"}(tab)
  out "Plot:  colors":cluster{"Freq out (Hz)":dbl[], dbl[]}[](graph)=[{"Freq out (Hz)"=[0.12, 0.157, 0.17, 0.2, 0.255, 0.3, 0.36, 0.43, 0.53, 0.62, 0.83, 1.13, 1.9, 3.1, 5.7], [0.5235452797399966, 0.29552092352028875, 0.2737421164710106, 0.21568813578812368, 0.1185839929679936, 0.08515276941439547, 0.06101183804371513, 0.04668629951754428, 0.035204330012184606, 0.03086203572346745, 0.023591124045179705, 0.020215154825776162, 0.018090572723952716, 0.019438138134990773, 0.01857318905405757]}, {"Freq out (Hz)"=[0.12, 0.157, 0.17, 0.2, 0.255, 0.3, 0.36, 0.43, 0.53, 0.62, 0.83, 1.13, 1.9, 3.1, 5.7], [0.0656135391669308, 0.054772440405347116, 0.0522629099950823, 0.04371088854633266, 0.03523285100342791, 0.02900111626314998, 0.025440548988990737, 0.02101121562555254, 0.021011523093336055, 0.019328530751225363, 0.014910006224862384, 0.014105227254331026, 0.013314780956190006, 0.013521019406290897, 0.01330461224529284]}, {"Freq out (Hz)"=[0.12, 0.157, 0.17, 0.2, 0.255, 0.3, 0.36, 0.43, 0.53, 0.62, 0.83, 1.13, 1.9, 3.1, 5.7], [0.09999999999999998, 0.07181400545085076, 0.06055403664621467, 0.044756474141397676, 0.03745802281585293, 0.0326046639929105, 0.030028053977987627, 0.027633142317063823, 0.025247316079283256, 0.023568572596915294, 0.019342950403538655, 0.01566092404315801, 0.010820835010041677, 0.007253169400547805, 0.003723860843753113]}, {"Freq out (Hz)"=[0.12, 0.157, 0.17, 0.2, 0.255, 0.3, 0.36, 0.43, 0.53, 0.62, 0.83, 1.13, 1.9, 3.1, 5.7], [0.42408311417676675, 0.24959376716905593, 0.15426970567966677, 0.09022254790421581, 0.03372450936284118, 0.016878763935177364, 0.01014073195520156, 0.005348477555273893, 0.0027186478751268037, 0.0017019666136308708, 0.0007529723868608053, 0.0005251370359167099, 0.00026555216651738116, 0.00015482483015247505, 8.482944249837319e-05]}, {"Freq out (Hz)"=[0.12, 0.157, 0.17, 0.2, 0.255, 0.3, 0.36, 0.43, 0.53, 0.62, 0.83, 1.13, 1.9, 3.1, 5.7], [0.000911255863194602, 0.0011036321553823387, 0.0010741443369011179, 0.0010497817854404558, 0.0014409222626060132, 0.0014435248453868136, 0.001895079686544743, 0.00209847764984426, 0.0030917275749309152, 0.003453790534096172, 0.0049004132317226005, 0.005447728357292778, 0.0053935404172149905, 0.00474657938472858, 0.004309703631596548]}]
  in  "parameter selectors":enum32{"Page 1"}(tab)
  in  "select B (T)":u16(ring)=8 items=["0.000", "5.000", "6.000", "7.000", "8.000", "9.000", "10.000", "11.000", "12.000"]
  in  "select θ (deg)":u16(ring)=2 items=["0.000", "30.000", "45.000", "60.000", "90.000"]
  in  "ignore T !":bool=TRUE
  in  "select T (K)":u16(ring)=10 items=["0.120", "0.127", "0.129", "0.140", "0.148", "0.150", "0.157", "0.160", "0.170", "0.179", "0.180", "0.197", "0.200", "0.220", "0.240", "0.249", "0.250", "0.255", "0.270", "0.280", "0.287", "0.300", "0.330", "0.360", "0.390", "0.400", "0.430", "0.480", "0.510", "0.512", "0.530", "0.580", "0.610", "0.620", "0.670", "0.680", "0.810", "0.830", "0.910", "1.000", "1.100", "1.120", "1.130", "1.230", "1.550", "1.800", "1.900", "1.970", "2.050", "3.000", "3.100", "3.150", "3.190", "3.310", "5.500", "5.700", "5.820", "6.000", "7.870", "9.800", "12.360", "14.800", "16.420", "18.040", "19.600"]
  in  "ignore B !":bool
  in  "ignore θ !":bool
  in  "X selector":T1=enum."T (K)"
  in  "select side (8S|4R)":i32(ring) items=["4000", "8000"]
  in  "ignore side !":bool
  in  "select change (1T|2B)":i32(ring) items=["1", "2"]
  in  "ignore change !":bool
  in  "constrained filenames":u16(ring) caption="files" items=["CeCoIn5_3rd_4026_ref_12T_0.127K_60deg_changeT_fsweep_labview_.dat", "CeCoIn5_3rd_40049_ref_12T_0.129K_60deg_changeT_fsweep_labview_.dat", "CeCoIn5_3rd_4027_ref_12T_0.15K_60deg_changeT_fsweep_labview_.dat", "CeCoIn5_3rd_4028_ref_12T_0.179K_60deg_changeT_fsweep_labview_.dat", "CeCoIn5_3rd_4029_ref_12T_0.20K_60deg_changeT_fsweep_labview_.dat", "CeCoIn5_3rd_4030_ref_12T_0.24K_60deg_changeT_fsweep_labview_.dat", "CeCoIn5_3rd_4031_ref_12T_0.287K_60deg_changeT_fsweep_labview_.dat", "CeCoIn5_3rd_4032_ref_12T_0.33K_60deg_changeT_fsweep_labview_.dat", "CeCoIn5_3rd_4033_ref_12T_0.43K_60deg_changeT_fsweep_labview_.dat", "CeCoIn5_3rd_4034_ref_12T_0.51K_60deg_changeT_fsweep_labview_.dat", "CeCoIn5_3rd_4035_ref_12T_0.62K_60deg_changeT_fsweep_labview_.dat", "CeCoIn5_3rd_4036_ref_12T_0.83K_60deg_changeT_fsweep_labview_.dat", "CeCoIn5_3rd_4037_ref_12T_1.13K_60deg_changeT_fsweep_labview_.dat", "CeCoIn5_3rd_4038_ref_12T_1.90K_60deg_changeT_fsweep_labview_.dat", "CeCoIn5_3rd_4039_ref_12T_3.15K_60deg_changeT_fsweep_labview_.dat", "CeCoIn5_3rd_4040_ref_12T_5.70K_60deg_changeT_fsweep_labview_.dat", "CeCoIn5_3rd_4041_ref_12T_7.87K_60deg_changeT_fsweep_labview_.dat", "CeCoIn5_3rd_4042_ref_12T_9.80K_60deg_changeT_fsweep_labview_.dat", "CeCoIn5_3rd_4043_ref_12T_12.36K_60deg_changeT_fsweep_labview_.dat", "CeCoIn5_3rd_4044_ref_12T_14.80K_60deg_changeT_fsweep_labview_.dat", "CeCoIn5_3rd_4045_ref_12T_16.42K_60deg_changeT_fsweep_labview_.dat", "CeCoIn5_3rd_4046_ref_12T_18.04K_60deg_changeT_fsweep_labview_.dat", "CeCoIn5_3rd_40047_ref_12T_19.60K_60deg_changeT_fsweep_labview_.dat"]
  in  "parameter selectors 2":enum32{"Page 1"}(tab)
  in  "colors":u32[](array[colorbox])=[7893503, 4390723, 2062078, 16740827, 16755712, 11121611, 8285330, 9272482, 9204890]
  in  "parameter":T1[](array[typedef])=[enum."ζ", enum."τ1", enum."τS", enum."τN", enum."τC", enum."κ0"]
  in  "parameter selectors 3":enum32{"Page 1"}(tab)
  out "file index":i32=40126
  out "T (K)":dbl=0.12 format="%#_10f"
  out "θ (deg)":dbl=45.0 format="%#_10f"
  out "B (T)":dbl=12.0
  in  "parameter selectors 5":enum32{"Page 1"}(tab)
  in  "Write τ's to  Math!":bool
  in  "Read  τ's  from  Math !":bool
  out "state of all selectors":map{T1, map{bool, dbl}}(c390)={enum."T (K)"={TRUE=0.18}, enum."B (T)"={FALSE=12.0}, enum."θ (deg)"={FALSE=45.0}, enum."side (S|R)"={FALSE=4000.0}, enum."change (B|T)"={FALSE=1.0}}
  out "state of all selectors string":string="__12T__45deg__4000side_"
  out "new selector names":map{T1, map{T4, string}}(c390)={enum."ζ"={enum."name"="ζ", enum."nameL"="zeta", enum."units"="sec", enum."prec"="%_4p"}, enum."τ1"={enum."name"="τ1", enum."nameL"="tau1", enum."units"="sec", enum."prec"="%_4p"}, enum."τS"={enum."name"="τS", enum."nameL"="tauS", enum."units"="sec", enum."prec"="%_4p"}, enum."τN"={enum."name"="τN", enum."nameL"="tauN", enum."units"="sec", enum."prec"="%_4p"}, enum."τC"={enum."name"="τC", enum."nameL"="tauC", enum."units"="sec", enum."prec"="%_4p"}, enum."κ0"={enum."name"="κ0", enum."nameL"="kappa0", enum."units"="WperK", enum."prec"="%_5p"}, enum."T (K)"={enum."name"="T", enum."nameL"="T", enum."units"="K", enum."prec"="%_4p"}, enum."B (T)"={enum."name"="B", enum."nameL"="B", enum."units"="T", enum."prec"="%_2p"}, enum."θ (deg)"={enum."name"="θ", enum."nameL"="theta", enum."units"="deg", enum."prec"="%_2p"}, enum."side (S|R)"={enum."name"="side", enum."nameL"="side", enum."units"="side", enum."prec"="%d"}}
  in  "parameters":enum32{"Page 1"}(tab)
  in  "ζ":dbl(slide)=0.5235452797399966 min=0.0 max=0.3 step=1e-06 scale=1e-05..1000.0 scale format="%#_3p"
  in  "T1":dbl(slide)=0.0656135391669308 min=0.0 max=0.3 step=1e-06 scale=0.0001..1000.0 scale format="%#_3p"
  in  "τS":dbl(slide)=0.09999999999999998 min=0.0 max=0.3 step=1e-06 scale=0.0001..10.0 scale format="%#_3p"
  in  "τN":dbl(slide)=0.42408311417676675 min=0.0 max=0.3 step=1e-06 scale=1e-06..1000.0 scale format="%#_3p"
  in  "τC":dbl(slide)=0.000911255863194602 min=0.0 max=0.3 step=1e-06 scale=0.0001..10.0 scale format="%#_3p"
  in  "κ0":dbl(slide)=4.1798641133515373e-10 min=0.0 max=0.3 step=1e-12 scale=1e-10..1e-06 scale format="%#_3p"
  in  "newton control":enum32{"Page 1", "Page 2"}(tab)
  in  "newton control":enum32{"Page 1"}(tab)
  in  "factor":dbl(slide)=0.01760532571594699 scale=1e-06..1.0 scale format="%#_3p"
  in  "# steps":i32=150
  out "goodness":dbl=0.0971098895063455 format="%#_3p"
  in  "parameter selectors 4":enum32{"Page 1"}(tab)
  in  "pause!":bool
  in  "go!":bool
  in  "weighting":T5=enum."dω √(|dz/dω|)"
  in  "newton action":T6=enum."onlygrads"
  out "logarithmic derivatives":dbl[](array[numeric])=[0.21766540771323906, 0.005013732582601321, -0.029033353202796715, -0.006766765617151386, -0.27927918821011405, -0.6583053657451554] format="%#_3g"
  in  "what":cluster{"scaling":dbl, "what":T1}[](array[cluster])=[{"scaling"=10.0, "what"=enum."ζ"}, {"scaling"=10.0, "what"=enum."τ1"}, {"scaling"=10.0, "what"=enum."τS"}, {"scaling"=10.0, "what"=enum."τN"}, {"scaling"=10.0, "what"=enum."τC"}, {"scaling"=1.0, "what"=enum."κ0"}]
  in  "newton pause":bool=TRUE
  in  "sweeper panel":T7(tab)
  out "Plot: sweep window":cluster{"Freq out (Hz)":dbl[], dbl[]}[](graph)
  in  "scale gauge: Plot: complex plane":dbl(slide)=2561121586.003556 min=0.0 max=0.3 step=1e-06 scale=3000000.0..100000000000.0 scale format="%#_3p"
  in  "ω0 (rad/sec)":dbl(slide)=140.85980015121274 scale=0.001..50000.0 scale format="%#_2p"
  in  "offset control tab":enum32{"Page 1"}(tab)
  in  "off\nRe\nIm":cluster{"Numeric":dbl, "Numeric":dbl}(slide)={"Numeric"=-112222222.22222222, "Numeric"=0.0} scale=-40000000.0..50000000.0 scale format="%#_1p"
  in  "cspan":dbl=0.003 format="%#_13g"
  in  "cursor window":T8={"left"=20184.313682072192, "right "=24669.14654231211, "center"=22426.730112192152, "window"=4484.832860239923, "cursors"=[0, 1, 2], "relative"=0, "absolute"=0, "fixed vertical offset"=0.0, "vertical offset"=0.0, "skew"=0.0, "default window frac"=0.1, "kind"=enum."symmetric", "skew.left"=0.5, "skew.right"=0.5, "Plot ref"=refnum, "wing order"=enum."forw"}
  in  "win":T9={"cen (Hz)"=23772.179970264126, "win (Hz)"=4484.832860239923, "left (Hz)"=21529.763540144166, "right (Hz)"=26014.596400384085}
  in  ":sweep is ON":bool
  in  "stopping criteria":T10={"function tolerance"=1e-06, "parameter tolerance"=1e-06, "max iterations"=100, "max function calls"=1000, "gradient tolerance"=1e-06, "max time (sec)"=-1.0}
  in  "uco! :u":bool
  out "cursor x selector":map{T1, dbl}(c390)={enum."T (K)"=0.12, enum."B (T)"=12.0, enum."θ (deg)"=45.0}
  in  "save data":enum32{"save/read"}(tab)
  in  "Save to file :s":bool
  in  "Freq sweep name template":T11={"prefix"="RuCl3-rod", "group"="f"}
  in  "Save folder":path=path "/opt/data"
  in  "freq sweep file name":string="f013_RuCl3-rod_082821.dat"
  in  "cursor index map":map{T1, i32}(c390)={enum."ζ"=0, enum."τ1"=1, enum."τS"=2, enum."τN"=3, enum."τC"=4, enum."κ0"=5, enum."m1"=6, enum."m2"=7, enum."m3"=8}
